vi "DataIn.vi"(8 "error in (no error)":errorcluster caption="错误输入（无错误）", 11 "XYPlot 输入":refnum<class "XYPlot.lvclass">) -> (0 "error out":errorcluster caption="错误输出", 1 "Data1":dbl[](array[numeric]), 2 "Data0":dbl[](array[numeric]), 3 "XYPlot 输出":refnum<class "XYPlot.lvclass">)   [LabVIEW 2018, in "DataDisplay.lvlib" / "XYPlot.lvclass"]
uses:
  XYPlot.lvclass
  XYPlot.lvclass/XYPlot.ctl
  DataDisplay.lvlib
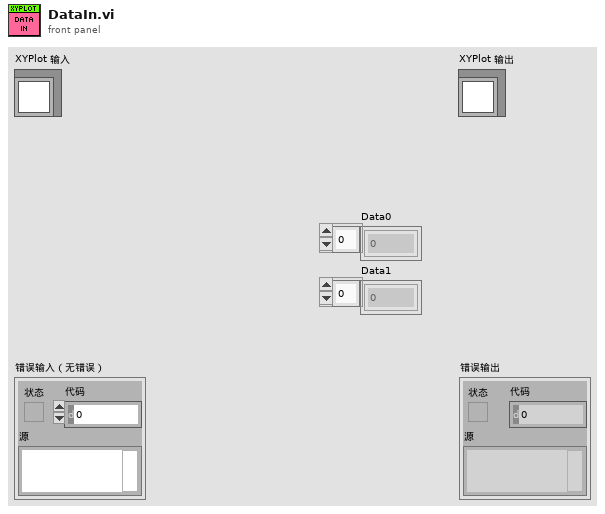
[diagram p1: front panel]
types:
  T1 = typedef "DataDisplay.lvlib/DD_DataStream.ctl" = cluster{"Data":dbl[]}[]
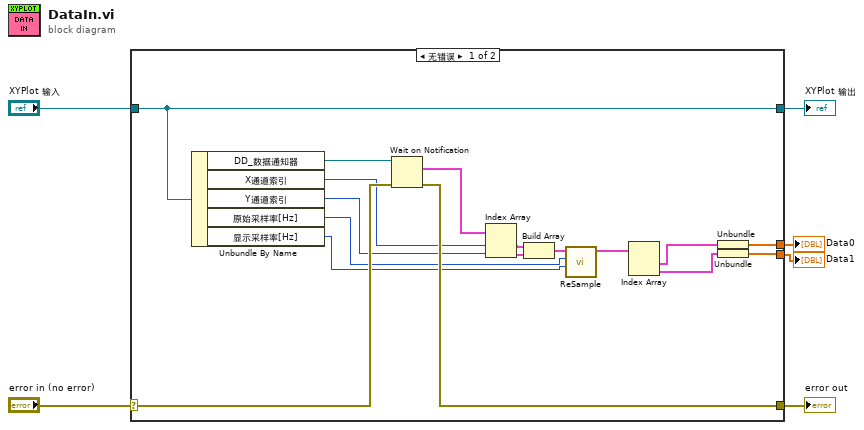
[diagram p0: block diagram]
diagram:
  n1 = case shown="无错误" "error in (no error)" {
    selector: "error in (no error)" -> [w20 w25]
    tunnel: [w19 w25] -> w5
    tunnel: [w23 w24] -> w3
    tunnel: "XYPlot 输入" -> [w23 w24]
    tunnel: [w16 _] -> w2
    tunnel: [w15 _] -> w1
    frame No Error {
      n2 = Unbundle By Name(w23) -> ("DD_数据通知器"=w21:refnum<notifier>, "X通道索引"=w18:i32, "Y通道索引"=w17:i32, "原始采样率[Hz]"=w8:i32, "显示采样率[Hz]"=w7:i32)
      n3 = Wait on Notification(notifier=w21, error in (no error)=w20) -> (notification=w22:T1, error out=w19:errorcluster)  [unwired: 2 in, 2 out]
      n4 = Index Array(array=w22, index #1=w18, index #2=w17) -> (element #1=w14:cluster{"Data":dbl[]}, element #2=w13:cluster{"Data":dbl[]})
      n5 = Build Array(w14, w13) -> (w12:cluster{"Data":dbl[]}[])
      n6 = call "ReSample.vi"("重采样率[Hz]"=w7, "原始采样率[Hz]"=w8, "原始数据"=w12) -> ("重采样后数据"=w11:cluster{dbl[]}[])  [unwired: 8 in]
      n7 = Index Array(array=w11) -> (element #1=w10:cluster{dbl[]}, element #2=w9:cluster{dbl[]})  [unwired: 2 in]
      n8 = Unbundle(w10) -> (w16:dbl[])
      n9 = Unbundle(w9) -> (w15:dbl[])
    }
    frame Error {
    }
  }
  "error out" <- w5
  "XYPlot 输出" <- w3
  "Data0" <- w2
  "Data1" <- w1
